vi "NichtlinearerRegler3.vi"(8 "Wgeschw.":dbl, 9 "Winkel":dbl, 10 "Geschwindigkeit":dbl, 11 "Weg":dbl) -> (2 "s? t:f":dbl)   [LabVIEW 2013]
uses:
  <vilib>/express/express arith-compare/Formula/XNode/ExpressFormulaBlockNode.xnode
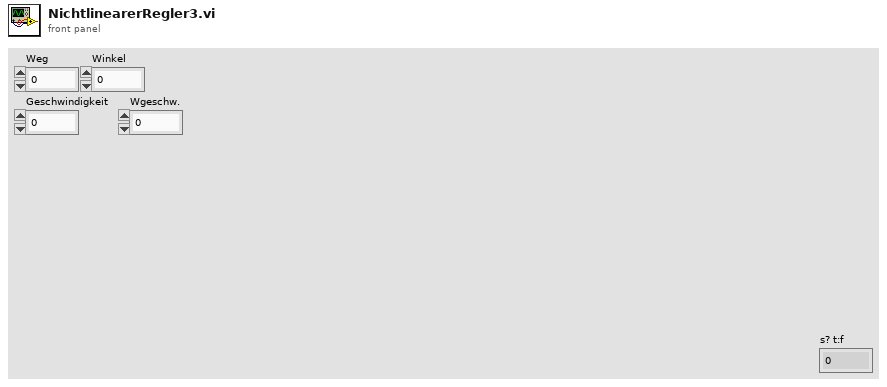
[diagram p1: front panel]
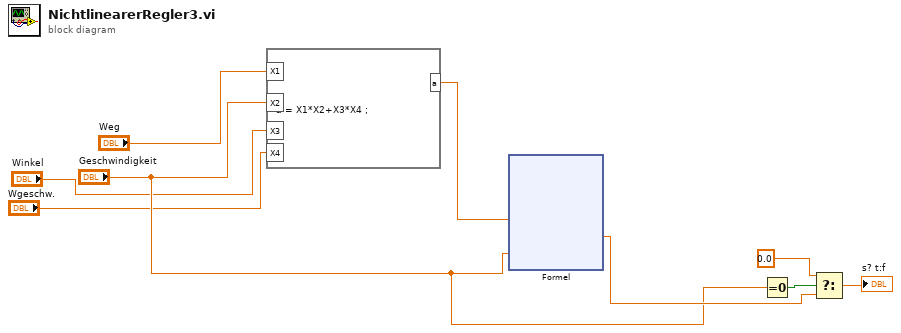
[diagram p0: block diagram]
diagram:
  n1 = formula code="a = X1*X2+X3*X4 ;"("X1"="Weg", "X2"="Geschwindigkeit", "X3"="Winkel", "X4"="Wgeschw.") -> ("a"=w4:dbl)
  n2 = xnode "Formel"("X1"=w4, "X2"="Geschwindigkeit") -> ("Ergebnis"=w6:dbl)  [unwired: 1 in, 1 out]
  n3 = Equal To 0? ("Gleich 0?")(x="Geschwindigkeit") -> (x = 0?=w9:bool)
  n4 = Select ("Auswählen")(t=0.0 ("value below threshold 2"), s=w9, f=w6) -> (s? t:f=→"s? t:f":dbl)
